vi "ECO_Query.vi"(0 "System no.":i32=1 min=1 step=1, 2 "Send":string, 5 "error in":errorcluster) -> (14 "Reply":string, 19 "error out":errorcluster)   [LabVIEW 2020]
doc: "Returns echo string. Reply should be equal to Send string."
panel:
  # "Returns echo string. Reply should be equal to Send string."
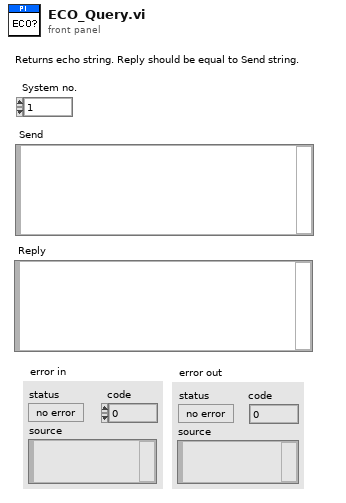
[diagram p1: front panel]
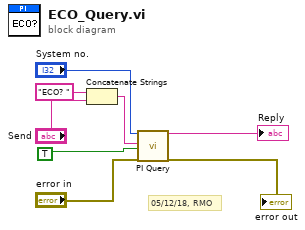
[diagram p0: block diagram]
diagram:
  # "05/12/18, RMO"
  n1 = Concatenate Strings("ECO? " ("string"), "Send") -> (w3:string)
  n2 = call "PI Query.vi"("System no."="System no.", "String to send"=w3, "Attach termination char.?"=TRUE ("Attach Linefeed?"), "error in"="error in") -> ("String read"=→"Reply":string, "error out"=→"error out":errorcluster)  [unwired: 3 in, 11 out]
